vi "time-sec-to-radian.vi"(1 "Numeric":dbl format="%<%H:%M:%S>t") -> (0 "radians":dbl format="%.10g")   [LabVIEW 2011]
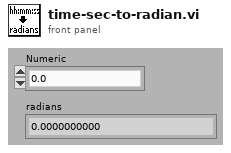
[diagram p1: front panel]
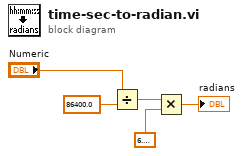
[diagram p0: block diagram]
diagram:
  n1 = Divide(x="Numeric", y=86400.0) -> (x/y=w3:dbl)
  n2 = Multiply(x=w3, y=6.283185307179586) -> (x*y=→"radians":dbl)
